vi "例10.2  利用高层函数采集单幅图像.vi"() -> ()   [LabVIEW 2017]
doc: "The Snap VI acquires an image and displays the image in an image control using low-level acquisition VIs. A snap is appropriate for low-speed or single-capture applications in which ease of programming is essential."
uses:
  <vilib>/userdefined/High Color/IMAQdx.ctl
  <vilib>/vision/driver/NI_Vision_Acquisition_Software.lvlib
panel:
  in  "Camera Name":T1
  out "Image":T2(plugin-control)
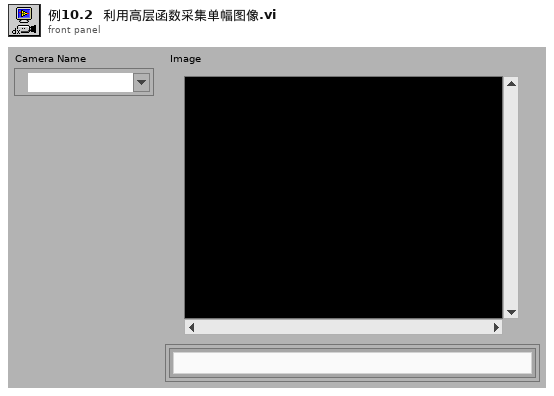
[diagram p1: front panel]
types:
  T1 = typedef "IMAQdx.ctl" = refnum<k21>
  T2 = typedef "IMAQ Image.ctl" = refnum<image>
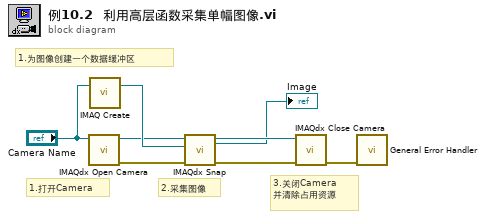
[diagram p0: block diagram]
diagram:
  # "1.为图像创建一个数据缓冲区"
  # "2.采集图像"
  # "3.关闭Camera\n并清除占用资源"
  # "1.打开Camera"
  n1 = call <vilib>:"IMAQdx Open Camera.vi"("Session In"="Camera Name") -> ("error out"=w1:errorcluster, "Session Out"=w5:T1)  [unwired: 2 in, 7 out]
  n2 = call "IMAQ Create"("Image Name"="Camera Name") -> ("New Image"=w7:T2)  [unwired: 3 in, 2 out]
  n3 = call <vilib>:"IMAQdx Snap.vi"("error in"=w1, "Image In"=w7, "Session In"=w5) -> ("error out"=w3:errorcluster, "Image Out"=→"Image":T2, "Session Out"=w8:T1)  [unwired: 6 out]
  n4 = call <vilib>:"IMAQdx Close Camera.vi"("error in"=w3, "Session In"=w8) -> ("error out"=w6:errorcluster)  [unwired: 9 out]
  n5 = call <vilib>:"General Error Handler.vi"("error in (no error)"=w6) -> ()  [unwired: 2 in, 13 out]
